vi "Glimpse set up to read sequence.vi"(0 "acquisition directory path":path, 3 "error in":errorcluster) -> (1 "Header2 file data out":T1, 4 "Header file data out":T2 {"Pixel depth" items=["8 bits", "16 bits", "Float", "Complex", "RGB", "HSL"]; "time of 1st frame, \nsec since 1/1/04" format="%.2f"}, 5 "acquisition directory path out":path=path "Glimpse set up to read sequence default value", 6 "Acquisition refnum array":refnum<file>[](array[refnum]), 7 "error out":errorcluster)   [LabVIEW 2016]
doc: "Opens the acquisition files and leaves them open. Opens the heaer file, reads it, and closes it. If there is an error, VI tries to close all open files before exiting."
uses:
  Header file data.ctl
  Seq file v 1/Offset table.ctl
  Seq file v 1/Offset.ctl
  Seq file v 1/file number.ctl
  Header2 file data.ctl
  GLIMPSE Globals.vi
panel:
  out "Number of acq files":i32
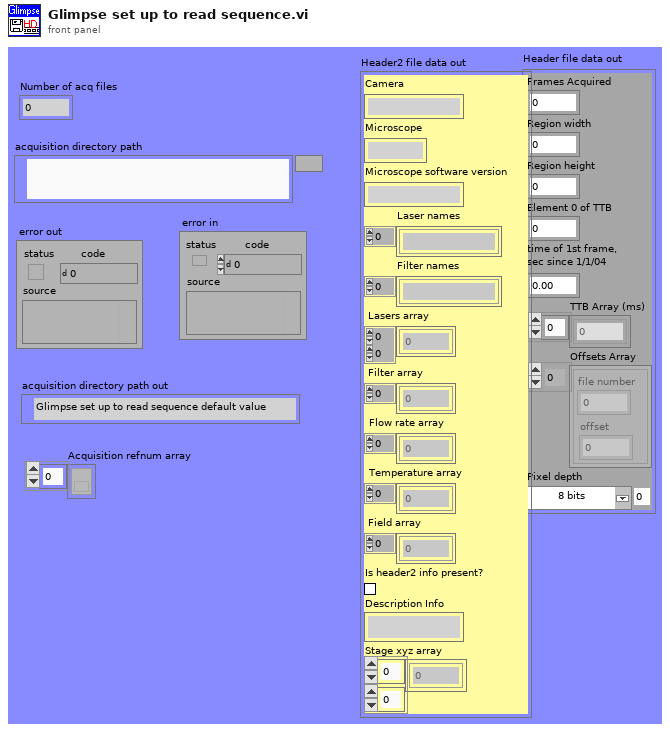
[diagram p1: front panel]
types:
  T1 = typedef "Header2 file data.ctl" = cluster{"Camera":string, "Microscope":string, "Microscope software version":string, "Laser names":string[], "Filter names":string[], "Lasers array":u16[][], "Filter array":u16[], "Flow rate array":dbl[], "Temperature array":dbl[], "Field array":u16[], "Is header2 info present?":bool, "Description Info":string, "Stage xyz array":dbl[][]}
  T2 = typedef "Header file data.ctl" = cluster{"Frames Acquired":u32, "Region width":i32, "Region height":i32, "Element 0 of TTB":u32, "time of 1st frame, \nsec since 1/1/04":dbl, "TTB Array (ms)":u32[], "Offsets Array":T3, "Pixel depth":u32}
  T3 = typedef "Offset table.ctl" = cluster{"offset":T4, "file number":T5}[]
  T4 = typedef "Offset.ctl" = i32
  T5 = typedef "file number.ctl" = u8
  T6 = enum16{"read/write", "read-only", "write-only", "write-only (truncate)"}
  T7 = enum16{"deny read/write", "deny write-only", "deny none"}
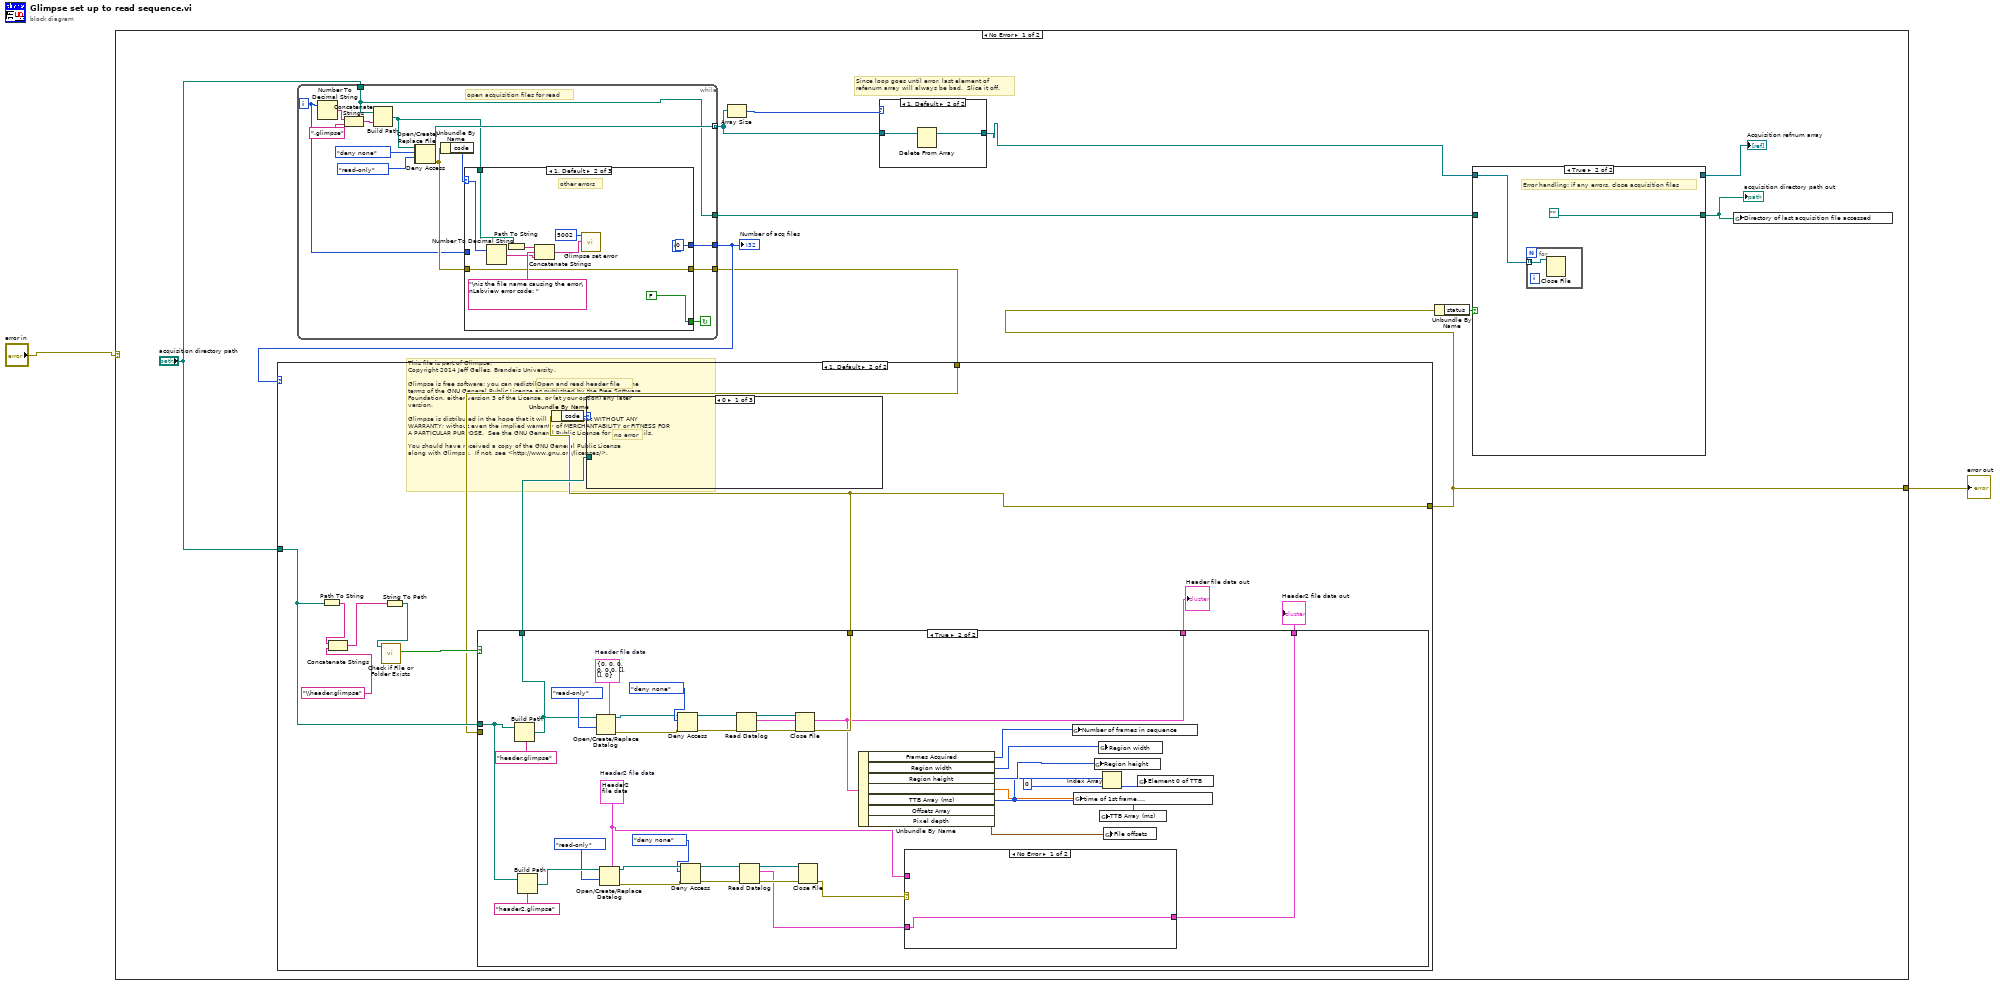
[diagram p0: block diagram]
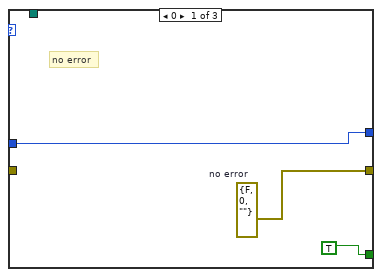
[diagram p4: hidden frame]
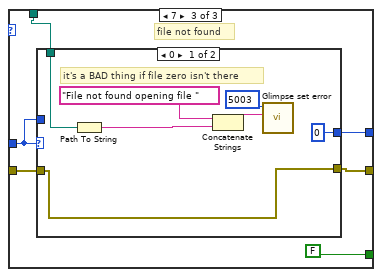
[diagram p5: hidden frame]
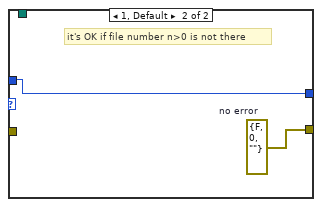
[diagram p6: hidden frame]
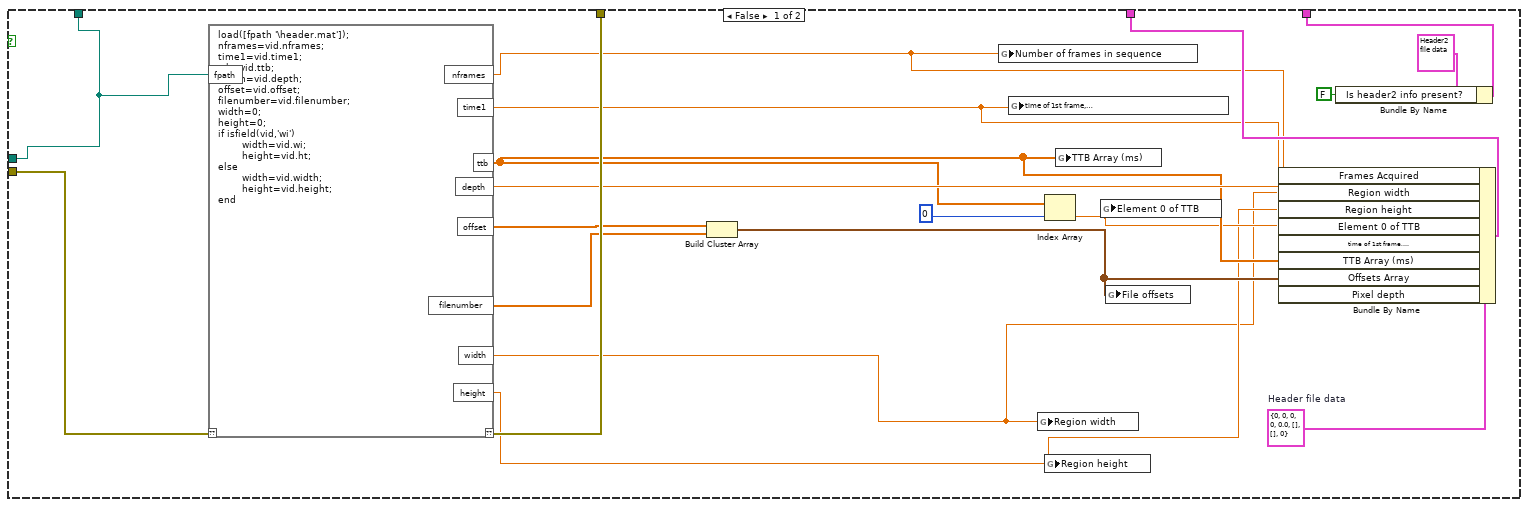
[diagram p8: hidden frame]
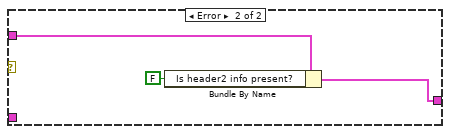
[diagram p9: hidden frame]
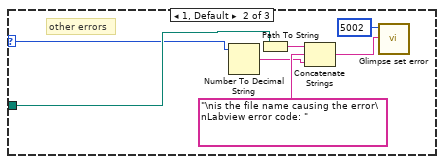
[diagram p10: hidden frame]
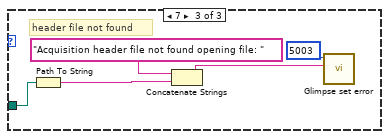
[diagram p11: hidden frame]
diagram:
  # "This file is part of Glimpse. \nCopyright 2014 Jeff Gelles, Brandeis University.    \n\nGlimpse is free software: you can redistribute it and/or modify it under the \nterms of the GNU General Public License as published by the Free Software \nFoundation, either version 3 of the License, or (at your option) any later \nversion.\n\nGlimpse is distributed in the hope that it will be useful, but WITHOUT ANY \nWARRANTY; without even the implied warranty of MERCHANTABILITY or FITNESS FOR \nA PARTICULAR PURPOSE.  See the GNU General Public License for more details.\n\nYou should have received a copy of the GNU General Public License\nalong with Glimpse.  If not, see <http://www.gnu.org/licenses/>."
  n1 = case shown="No Error" "error in" {
    selector: "error in" -> [_ w149]
    tunnel: [w4 w149] -> w2
    frame No Error {
      # "Since loop goes until error, last element of\nrefenum array will always be bad.  Slice it off."
      n2 = while {
        tunnel: "acquisition directory path" -> [w24]
        tunnel: [w24] -> w8
        tunnel: [w29] -> w13
        tunnel: [w27] -> w9 mode=indexing
        tunnel: [w26] -> w12
        i -> [w30]
        stop <- w28 continue-if-true
        # "open acquisition files for read"
        n3 = Number To Decimal String(number=w30) -> (decimal integer string=w37:string)  [unwired: 1 out]
        n4 = Concatenate Strings(w37, ".glimpse" ("string")) -> (w35:string)
        n5 = Build Path(base path=w24, name or relative path=w35) -> (appended path=w25:path)
        n6 = Open/Create/Replace File(file path (use dialog)=w25, access (0:read/write)=T6."read-only" ("open mode (0)")) -> (refnum out=w22:refnum<file>, error out=w23:errorcluster)  [unwired: 1 in, 4 out]
        n7 = Deny Access(4:w23, 6:T7."deny none" ("deny mode (2)"), 7:w22) -> (0:w31:errorcluster, 3:w27:refnum<file>)
        n8 = Unbundle By Name(w31) -> ("code"=w32:i32)
        n9 = case shown="1, Default" w32 {
          selector: w32 -> [_ w41 _]
          tunnel: w31 -> [_ w45 w52]
          tunnel: w25 -> [_ w50 w54]
          tunnel: w30 -> [w40 _ w56]
          tunnel: [w40 0 w55] -> w29
          tunnel: [TRUE FALSE FALSE] -> w28
          tunnel: [w38 w45 w51] -> w26
          frame 0 {
            w38 = errorcluster {"status"=FALSE, "code"=0, "source"=""}  # no error
            # "no error"
          }
          frame 1, Default {
            (unwired) 0
            # "other errors"
            n10 = Number To Decimal String(number=w41) -> (decimal integer string=w43:string)  [unwired: 1 out]
            n11 = Path To String(path=w50) -> (string=w47:string)
            n12 = Concatenate Strings(w47, "\nis the file name causing the error\nLabview error code: " ("string"), w43) -> (w42:string)
            n13 = call "Glimpse set error.vi"("code"=5002, "Additional information"=w42) -> ()  [unwired: 1 in, 6 out]
          }
          frame 7 {
            # "file not found"
            n14 = case shown="0" w56 {
              tunnel: w56 -> [_ w65]
              tunnel: [0 w65] -> w55
              tunnel: w54 -> [w60 _]
              tunnel: [w59 w64] -> w51
              tunnel: w52 -> [w59 _]
              frame 0 {
                # "it's a BAD thing if file zero isn't there"
                n15 = Path To String(path=w60) -> (string=w62:string)
                n16 = Concatenate Strings("File not found opening file " ("string"), w62) -> (w57:string)
                n17 = call "Glimpse set error.vi"("code"=5003, "Additional information"=w57) -> ()  [unwired: 1 in, 6 out]
              }
              frame 1, Default {
                w64 = errorcluster {"status"=FALSE, "code"=0, "source"=""}  # no error
                # "it's OK if file number n>0 is not there"
              }
            }
          }
        }
      }
      "Number of acq files" <- w13
      n18 = case shown="1, Default" w13 {
        tunnel: [w66 w69] -> w4
        tunnel: w12 -> [w66 w70]
        tunnel: "acquisition directory path" -> [_ w72]
        frame 0 {
        }
        frame 1, Default {
          # "Open and read header file"
          n19 = Path To String(path=w72) -> (string=w76:string)
          n20 = Concatenate Strings(w76, "\\header.glimpse" ("search string")) -> (w74:string)
          n21 = String To Path(string=w74) -> (path=w77:path)
          n22 = call <vilib>:"Check if File or Folder Exists.vi"("path"=w77) -> ("file or folder exists?"=w73:bool)  [unwired: 1 in, 9 out]
          n23 = case shown="True" w73 {
            tunnel: w72 -> [w94 w102]
            tunnel: [w94 w129] -> w71
            tunnel: w70 -> [w96 _]
            tunnel: [w95 w116] -> w69
            tunnel: [w92 w113] -> w68
            tunnel: [w79 w98] -> w67
            frame False {
              w93 = T2 {"Frames Acquired"=0, "Region width"=0, "Region height"=0, "Element 0 of TTB"=0, "time of 1st frame, \nsec since 1/1/04"=0.0, "TTB Array (ms)"=[], "Offsets Array"=[], "Pixel depth"=0}  # Header file data
              n24 = script code="load([fpath '\\header.mat']);\nnframes=vid.nframes;\ntime1=vid.time1;\nttb=vid.ttb;\ndepth=vid.depth;\noffset=vid.offset;\nfilenumber=vid.filenumber;\nwidth=0;\nheight=0;\nif isfield(vid,'wi')\n        width=vid.wi;\n        height=vid.ht;\nelse\n        width=vid.width;\n        height=vid.height;\nend"("??"=w96, "fpath"=w94) -> ("??"=w95:errorcluster, "nframes"=w84:dbl, "time1"=w88:dbl, "ttb"=w89:dbl[], "offset"=w82:dbl[], "filenumber"=w83:dbl[], "width"=w85:dbl, "height"=w86:dbl, "depth"=w91:dbl)
              n25 = Build Cluster Array(w82, w83) -> (w90:cluster{dbl, dbl}[])
              n26 = global write "GLIMPSE Globals.vi" "Number of frames in sequence"(w84) -> ()
              n27 = global write "GLIMPSE Globals.vi" "time of 1st frame, \nsec since 1/1/04"(w88) -> ()
              n28 = global write "GLIMPSE Globals.vi" "Region width"(w85) -> ()
              n29 = Index Array(array=w89, index=0) -> (element=w87:dbl)
              n30 = global write "GLIMPSE Globals.vi" "Region height"(w86) -> ()
              n31 = global write "GLIMPSE Globals.vi" "TTB Array (ms)"(w89) -> ()
              n32 = global write "GLIMPSE Globals.vi" "Element 0 of TTB"(w87) -> ()
              n33 = global write "GLIMPSE Globals.vi" "File offsets"(w90) -> ()
              n34 = Bundle By Name(cluster=w93, "Frames Acquired"=w84, "Region width"=w85, "Region height"=w86, "Element 0 of TTB"=w87, "time of 1st frame, \nsec since 1/1/04"=w88, "TTB Array (ms)"=w89, "Offsets Array"=w90, "Pixel depth"=w91) -> (w92:T2)
              n35 = Bundle By Name(cluster=T1 {"Camera"="", "Microscope"="", "Microscope software version"="", "Laser names"=[], "Filter names"=[], "Lasers array"=[], "Filter array"=[], "Flow rate array"=[], "Temperature array"=[], "Field array"=[], "Is header2 info present?"=FALSE, "Description Info"="", "Stage xyz array"=[]} ("input cluster"), "Is header2 info present?"=FALSE) -> (w79:T1)
            }
            frame True {
              w99 = T1 {"Camera"="", "Microscope"="", "Microscope software version"="", "Laser names"=[], "Filter names"=[], "Lasers array"=[], "Filter array"=[], "Flow rate array"=[], "Temperature array"=[], "Field array"=[], "Is header2 info present?"=FALSE, "Description Info"="", "Stage xyz array"=[]}  # Header2 file data
              w131 = T2 {"Frames Acquired"=0, "Region width"=0, "Region height"=0, "Element 0 of TTB"=0, "time of 1st frame, \nsec since 1/1/04"=0.0, "TTB Array (ms)"=[], "Offsets Array"=[], "Pixel depth"=0}  # Header file data
              n36 = Build Path(base path=w102, name or relative path="header.glimpse" ("search string")) -> (appended path=w129:path)
              n37 = Build Path(base path=w102, name or relative path="header2.glimpse" ("search string")) -> (appended path=w105:path)
              n38 = Open/Create/Replace Datalog(5:w131, 9:T6."read-only" ("open mode (0)"), 11:w129) -> (0:w114:errorcluster, 3:w115:refnum<k1>)  [unwired: 1 in, 3 out]
              n39 = Open/Create/Replace Datalog(5:w99, 9:T6."read-only" ("open mode (0)"), 11:w105) -> (0:w112:errorcluster, 3:w111:refnum<k1>)  [unwired: 1 in, 3 out]
              n40 = Deny Access(4:w114, 6:T7."deny none" ("deny mode (2)"), 7:w115) -> (0:w127:errorcluster, 3:w126:refnum<k1>)
              n41 = Deny Access(4:w112, 6:T7."deny none" ("deny mode (2)"), 7:w111) -> (0:w107:errorcluster, 3:w108:refnum<k1>)
              n42 = Read Datalog(4:w127, 7:w126) -> (0:w116:errorcluster, 2:w113:T2, 3:w125:refnum<k1>)  [unwired: 1 out]
              n43 = Read Datalog(4:w107, 7:w108) -> (0:w110:errorcluster, 2:w100:T1, 3:w109:refnum<k1>)  [unwired: 1 out]
              n44 = Close File(refnum=w125, error in=w116) -> ()  [unwired: 2 out]
              n45 = Close File(refnum=w109, error in=w110) -> (error out=w101:errorcluster)  [unwired: 1 out]
              n46 = Unbundle By Name(w113) -> ("Frames Acquired"=w124:u32, "Region width"=w123:i32, "Region height"=w122:i32, "time of 1st frame, \nsec since 1/1/04"=w121:dbl, "TTB Array (ms)"=w118:u32[], "Offsets Array"=w120:T3)  [unwired: 1 out]
              n47 = case shown="No Error" w101 {
                tunnel: w100 -> [w133 _]
                tunnel: w99 -> [_ w136]
                tunnel: [w133 w135] -> w98
                frame No Error {
                }
                frame Error {
                  n48 = Bundle By Name(cluster=w136, "Is header2 info present?"=FALSE) -> (w135:T1)
                }
              }
              n49 = global write "GLIMPSE Globals.vi" "Number of frames in sequence"(w124) -> ()
              n50 = global write "GLIMPSE Globals.vi" "time of 1st frame, \nsec since 1/1/04"(w121) -> ()
              n51 = global write "GLIMPSE Globals.vi" "Region height"(w122) -> ()
              n52 = global write "GLIMPSE Globals.vi" "Region width"(w123) -> ()
              n53 = global write "GLIMPSE Globals.vi" "TTB Array (ms)"(w118) -> ()
              n54 = Index Array(array=w118, index=0) -> (element=w119:u32)
              n55 = global write "GLIMPSE Globals.vi" "File offsets"(w120) -> ()
              n56 = global write "GLIMPSE Globals.vi" "Element 0 of TTB"(w119) -> ()
            }
          }
          "Header file data out" <- w68
          "Header2 file data out" <- w67
          n57 = Unbundle By Name(w69) -> ("code"=w78:i32)
          n58 = case shown="0" w78 {
            selector: w78 -> [_ w137 _]
            tunnel: w71 -> [_ w138 w146]
            frame 0 {
              # "no error"
            }
            frame 1, Default {
              # "other errors"
              n59 = Number To Decimal String(number=w137) -> (decimal integer string=w140:string)  [unwired: 1 out]
              n60 = Path To String(path=w138) -> (string=w143:string)
              n61 = Concatenate Strings(w143, "\nis the file name causing the error\nLabview error code: " ("string"), w140) -> (w139:string)
              n62 = call "Glimpse set error.vi"("code"=5002, "Additional information"=w139) -> ()  [unwired: 1 in, 6 out]
            }
            frame 7 {
              # "header file not found"
              n63 = Path To String(path=w146) -> (string=w147:string)
              n64 = Concatenate Strings("Acquisition header file not found opening file: " ("string"), w147) -> (w144:string)
              n65 = call "Glimpse set error.vi"("code"=5003, "Additional information"=w144) -> ()  [unwired: 1 in, 6 out]
            }
          }
        }
      }
      n66 = Array Size(array=w9) -> (size(s)=w10:i32)
      n67 = case shown="1, Default" w10 {
        tunnel: w9 -> [w19 w21]
        tunnel: [w19 w20] -> w5
        frame 0 {
        }
        frame 1, Default {
          n68 = Delete From Array(array=w21) -> (array with subset deleted=w20:refnum<file>[])  [unwired: 2 in, 1 out]
        }
      }
      n69 = Unbundle By Name(w4) -> ("status"=w3:bool)
      n70 = case shown="True" w3 {
        tunnel: w8 -> [w15 _]
        tunnel: [w15 path ""] -> w7
        tunnel: [w14 _] -> w6
        tunnel: w5 -> [w14 w16]
        frame False {
          # "no errors"
        }
        frame True {
          # "Error handling: if any errors, close acquisition files"
          n71 = for {
            tunnel: w16 -> [w18] mode=indexing
            n72 = Close File(refnum=w18) -> ()  [unwired: 1 in, 2 out]
          }
        }
      }
      "acquisition directory path out" <- w7
      "Acquisition refnum array" <- w6
      n73 = global write "GLIMPSE Globals.vi" "Directory of last acquisition file accessed"(w7) -> ()
    }
    frame Error {
    }
  }
  "error out" <- w2
